vi "Test Sweep.vi"(8 "error in (no error)":errorcluster, 11 "LockinDAQ in":refnum<class "LockinDAQ.lvclass">=refnum) -> (0 "error out":errorcluster, 3 "LockinDAQ out":refnum<class "LockinDAQ.lvclass">)   [LabVIEW 2016, in "Lockin.DAQ.lvclass"]
uses:
  Lockin.DAQ.lvclass
  <vilib>/Analysis/NI_AALBase.lvlib
  Typedefs/REF-cluster.ctl
  <vilib>/Analysis/baseanly.llb/Mean (DBL).vi
  Typedefs/Function-enum.ctl
  Typedefs/AO-cluster.ctl
  Waveguide Model/Waveguide Model--Cluster.ctl
  Typedefs/Sampling.ctl
panel:
  in  "sampling":T1={"Fs"=204789.0, "#s"=15753}
  in  "Enum":enum16{"X", "Y", "R", "Theta", "Mean"}(ring)
  in  "No. Lockins":i32=1 min=1
  in  "stop":bool
  in  "Simulate Waveguide":bool
  out "Average time (ms)":dbl=0.328125
  in  "Waveguide Cluster":T2
  out "Waveform Chart 2":u32(graph)
  in  "Channels: Lockin":T3={"Ch"=[1], " f (Hz)"=[13.0], "Phase (°)"=[0.0], "TC (s)"=[0.1], "order"=[1]} {"order" min=1; "TC (s)" min=0.0001 format="%#_3p"; "Phase (°)" format="%.3g"; "f (Hz)" format="%.3g"}
  out "Waveform Chart":dbl[][](graph)=[[-0.22911635604378638]]
  in  "AO Chanels":T4={"Ch"=[0], "Amp (V)"=[0.01], "DC (V)"=[0.0], "f (Hz)"=[13.0], "Phase (°)"=[0.0], "Function"=[enum."Sine"], "Sweep?"=[FALSE]} {"f (Hz)" min=0.001 max=10000.0 format="%.3g"; "Phase (°)" format="%.3g"; "DC (V)" format="%.3p"; "Amp (V)" min=0.0 max=10.0 format="%.3p"}
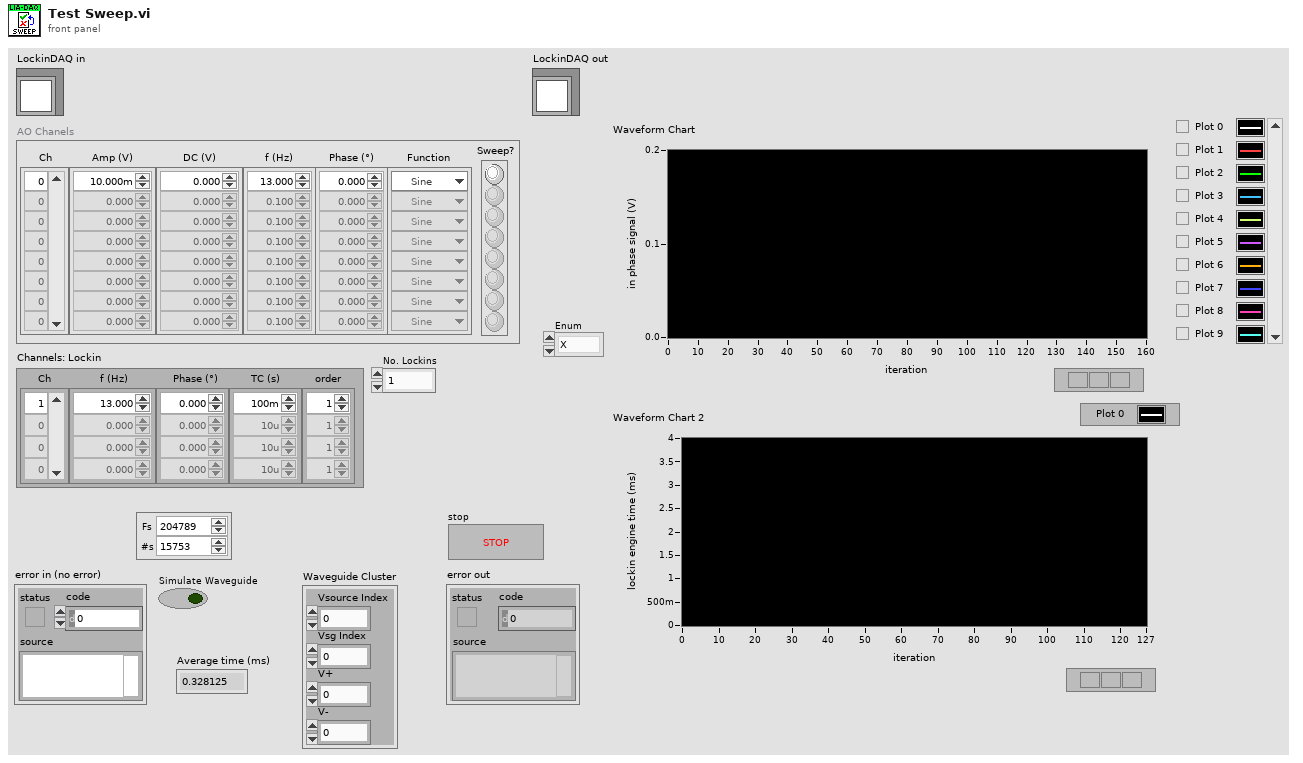
[diagram p1: front panel]
types:
  T1 = typedef "Lockin.DAQ.lvclass/Sampling.ctl" = cluster{"Fs":dbl, "#s":i32}
  T2 = typedef "Lockin.DAQ.lvclass/Waveguide Model--Cluster.ctl" = cluster{"Vsource Index":i32, "Vsg Index":i32, "V+":i32, "V-":i32}
  T3 = typedef "Lockin.DAQ.lvclass/REF-cluster.ctl" = cluster{"Ch":i32[], " f (Hz)":dbl[], "Phase (°)":dbl[], "TC (s)":dbl[], "order":i32[]}
  T4 = typedef "Lockin.DAQ.lvclass/AO-cluster.ctl" = cluster{"Ch":i32[], "Amp (V)":dbl[], "DC (V)":dbl[], "f (Hz)":dbl[], "Phase (°)":dbl[], "Function":T5[], "Sweep?":bool[]}
  T5 = typedef "Lockin.DAQ.lvclass/Function-enum.ctl" = enum16{"Sine", "Triangle", "Square", "Sawtooth"}
  T6 = typedef "Lockin.DAQ.lvclass/Results--Cluster.ctl" = cluster{"Time Stamp":timestamp, "Results":dbl[][]}
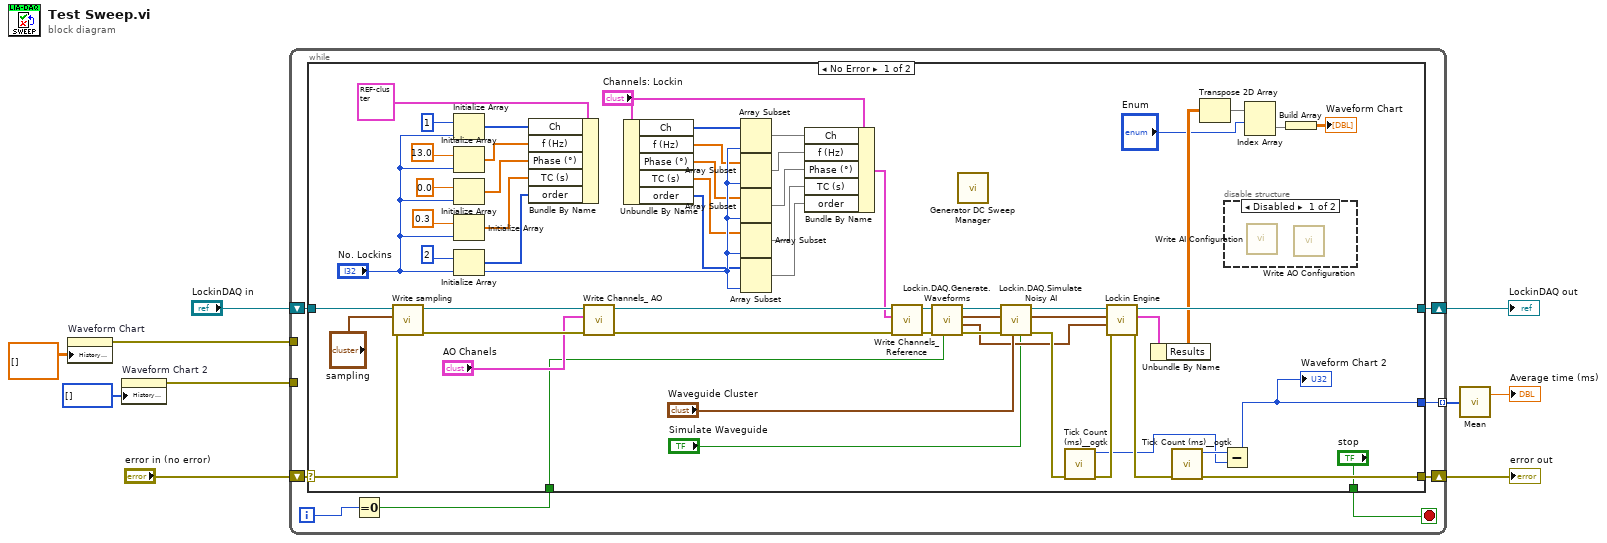
[diagram p0: block diagram]
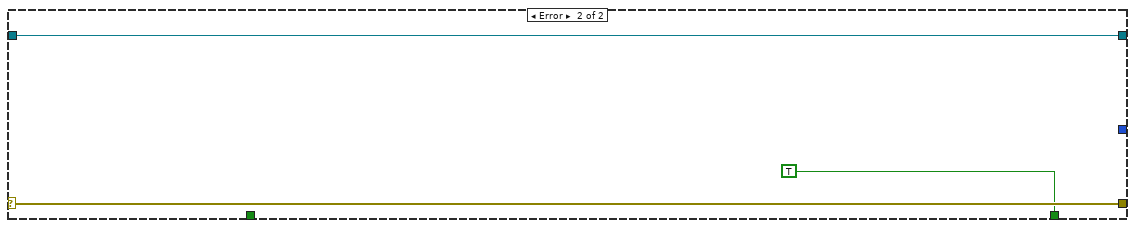
[diagram p3: hidden frame]
diagram:
  n1 = property on="Waveform Chart" class="WFChart (strict)"("History Data"=dbl[][] []) -> (error out=w2:errorcluster)  [unwired: 2 in, 1 out]
  n2 = property on="Waveform Chart 2" class="WFChart (strict)"("History Data"=u32[] []) -> (error out=w3:errorcluster)  [unwired: 2 in, 1 out]
  n3 = while {
    shift-right: [w17] -> w9
    shift-left: "error in (no error)" -> [w18]
    shift-right: [w15] -> w7
    shift-left: "LockinDAQ in" -> [w16]
    tunnel: [w14] -> w4 mode=indexing
    tunnel: w3 -> [_]
    tunnel: w2 -> [_]
    i -> [w12]
    stop <- w11 stop-if-true
    n4 = Equal To 0?(x=w12) -> (x = 0?=w13:bool)
    n5 = case shown="No Error" w18 {
      selector: w18 -> [w72 w79]
      tunnel: [w59 w79] -> w17
      tunnel: [w68 w78] -> w15
      tunnel: w16 -> [w73 w78]
      tunnel: [w57 _] -> w14
      tunnel: w13 -> [w52 _]
      tunnel: ["stop" TRUE ("stop")] -> w11
      frame No Error {
        n6 = call "Write sampling.vi"("error in (no error)"=w72, "sampling"="sampling", "LockinDAQ"=w73) -> ("error out"=w64:errorcluster, "LockinDAQ out"=w65:refnum<class "LockinDAQ.lvclass">)  [unwired: 7 in]
        n7 = Initialize Array(1, "No. Lockins") -> (w36:i32[])
        n8 = Initialize Array(13.0, "No. Lockins") -> (w37:dbl[])
        n9 = Initialize Array(0.0, "No. Lockins") -> (w38:dbl[])
        n10 = Initialize Array(0.3, "No. Lockins") -> (w39:dbl[])
        n11 = Initialize Array(2, "No. Lockins") -> (w40:i32[])
        n12 = Bundle By Name(cluster=T3 {"Ch"=[1], " f (Hz)"=[13.0], "Phase (°)"=[0.0], "TC (s)"=[0.3], "order"=[1]} ("Channels: Lockin"), "Ch"=w36, "f (Hz)"=w37, "Phase (°)"=w38, "TC (s)"=w39, "order"=w40) -> ()  [unwired: 1 out]
        n13 = call "Write Channels_ AO.vi"("error in (no error)"=w64, "Channels: AO"="AO Chanels", "LockinDAQ"=w65) -> ("error out"=w66:errorcluster, "LockinDAQ out"=w67:refnum<class "LockinDAQ.lvclass">)  [unwired: 7 in]
        n14 = Unbundle By Name("Channels: Lockin") -> ("Ch"=w32:i32[], "f (Hz)"=w22:dbl[], "Phase (°)"=w23:dbl[], "TC (s)"=w24:dbl[], "order"=w25:i32[])
        n15 = Array Subset(array=w32, length="No. Lockins") -> (w31:i32[])  [unwired: 1 in]
        n16 = Array Subset(array=w22, length="No. Lockins") -> (w21:dbl[])  [unwired: 1 in]
        n17 = Array Subset(array=w23, length="No. Lockins") -> (w26:dbl[])  [unwired: 1 in]
        n18 = Array Subset(array=w24, length="No. Lockins") -> (w27:dbl[])  [unwired: 1 in]
        n19 = Array Subset(array=w25, length="No. Lockins") -> (w28:i32[])  [unwired: 1 in]
        n20 = Bundle By Name(cluster="Channels: Lockin", "Ch"=w31, "f (Hz)"=w21, "Phase (°)"=w26, "TC (s)"=w27, "order"=w28) -> (w20:T3)
        n21 = call "Write Channels_ Reference.vi"("error in (no error)"=w66, "Channels: Lockin"=w20, "LockinDAQ"=w67) -> ("error out"=w49:errorcluster, "LockinDAQ out"=w48:refnum<class "LockinDAQ.lvclass">)  [unwired: 7 in]
        n22 = call "Lockin.DAQ.Generate.Waveforms.vi"("Reset?"=w52, "error in (no error)"=w49, "LockinDAQ"=w48) -> ("error out"=w74:errorcluster, "REF []"=w51:waveform(dbl)[], "AO []"=w76:waveform(dbl)[], "LockinDAQ out"=w75:refnum<class "LockinDAQ.lvclass">)  [unwired: 4 in, 1 out]
        n23 = call "Generator DC Sweep Manager.vi"() -> ()  [unwired: 8 in, 4 out]
        n24 = call "Lockin.DAQ.Simulate Noisy AI.vi"("Simulate Waveguide [T]"="Simulate Waveguide", "Waveguide Cluster"="Waveguide Cluster", "error in (no error)"=w74, "AO []"=w76, "LockinDAQ"=w75) -> ("error out"=w61:errorcluster, "Noisy AI []"=w71:waveform(dbl)[], "LockinDAQ out"=w70:refnum<class "LockinDAQ.lvclass">)  [unwired: 4 in]
        n25 = call <userlib>:"Tick Count (ms)__ogtk.vi"("error in (no error)"=w61) -> ("error out"=w60:errorcluster, "millisecond timer value"=w19:u32)  [unwired: 9 in]
        n26 = call "Lockin Engine.vi"("error in (no error)"=w60, "REF Waveforms"=w51, "AI Waveforms"=w71, "LockinDAQ"=w70) -> ("error out"=w56:errorcluster, "Averaged Results (X,Y,R,Theta,Mean)"=w62:T6, "LockinDAQ out"=w68:refnum<class "LockinDAQ.lvclass">)  [unwired: 4 in, 1 out]
        n27 = Unbundle By Name(w62) -> ("Results"=w35:dbl[][])
        n28 = call <userlib>:"Tick Count (ms)__ogtk.vi"("error in (no error)"=w56) -> ("error out"=w59:errorcluster, "millisecond timer value"=w58:u32)  [unwired: 9 in]
        n29 = Transpose 2D Array(2D array=w35) -> (transposed array=w69:dbl[][])
        n30 = Subtract(x=w58, y=w19) -> (x-y=w57:u32)
        "Waveform Chart 2" <- w57
        n31 = disable-structure shown="Disabled" {
          frame Disabled {
            n32 = call "Write AI Configuration.vi"() -> ()  [unwired: 10 in, 2 out]
            n33 = call "Write AO Configuration.vi"() -> ()  [unwired: 10 in, 2 out]
          }
          frame Enabled {
          }
        }
        n34 = Index Array(array=w69, index (row)="Enum") -> (element=w54:dbl[])  [unwired: 1 in]
        n35 = Build Array(w54) -> (→"Waveform Chart":dbl[][])
      }
      frame Error {
      }
    }
  }
  "error out" <- w9
  "LockinDAQ out" <- w7
  n36 = call-poly <vilib>:"Mean.vi"("X"=w4) -> ("mean"=→"Average time (ms)":dbl)  [unwired: 1 out]
